vi "PC_TDVM_Single.vi"() -> ()   [LabVIEW 2021]
uses:
  Time Domain Measurement/Typedefs/Time Domain Measurements.ctl
  Time Domain Measurement/Typedefs/Timing & Trigger Settings.ctl
  Time Domain Measurement/Typedefs/Timing Settings.ctl
  Time Domain Measurement/Typedefs/Trigger Settings.ctl
  Time Domain Measurement/DAQ_Time Domain Measurement.lvlib
panel:
  out "Time Domain Measurements":T1={"Mean DC Voltage (V)"=[1.1069459616870432], "Vpp Amplitude(V)"=[5.075915353058466], "Voltage Frequency(Hz)"=[101.01007488404397], "Voltage Waveform Period (s)"=[0.009900002560615512], "Voltage Waveform duty cycle (%)"=[22.01996744294479]} {"Voltage Waveform duty cycle (%)" format="%.2p"; "Voltage Waveform Period (s)" format="%.2p"; "Voltage Frequency(Hz)" format="%.2p"; "Vpp Amplitude(V)" format="%.2p"; "Mean DC Voltage (V)" format="%.2p"}
  out "error out":errorcluster
  out "Voltage Waveforms":waveform(dbl)[](graph)=[{"t0"=timestamp(3797419317.779368 s since 1904-01-01), "dt"=9.999999999999972e-06, "Y"=array[10000 elements], "attributes"=variant("NI_ChannelName"=variant(string "Dev1/ai2"), "NI_UnitDescription"=variant(string "Volts"))}]
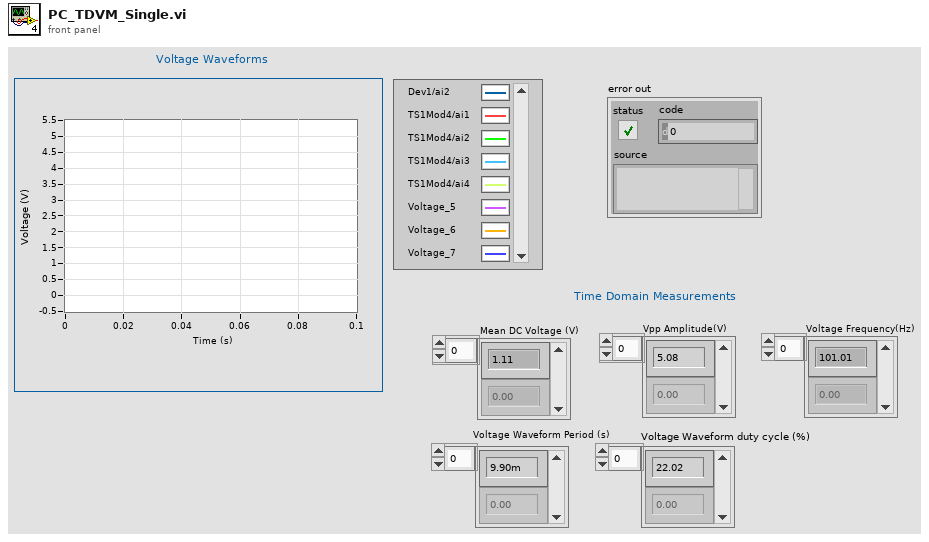
[diagram p1: front panel]
types:
  T1 = typedef "DAQ_Time Domain Measurement.lvlib/Time Domain Measurements.ctl" = cluster{"Mean DC Voltage (V)":dbl[], "Vpp Amplitude(V)":dbl[], "Voltage Frequency(Hz)":dbl[], "Voltage Waveform Period (s)":dbl[], "Voltage Waveform duty cycle (%)":dbl[]}
  T2 = typedef "DAQ_Time Domain Measurement.lvlib/Timing & Trigger Settings.ctl" = cluster{"Timing Settings":T3, "Trigger Settings":T4}
  T3 = typedef "DAQ_Time Domain Measurement.lvlib/Timing Settings.ctl" = cluster{"Sample Clock Source":tag, "Sample Rate(Hz)":dbl, "Number of Samples":i32, "Sample Timing Engine":enum16{"te0", "te1", "ai", "Auto"}}
  T4 = typedef "DAQ_Time Domain Measurement.lvlib/Trigger Settings.ctl" = cluster{"Trigger Type":enum16{"No Trigger", "Digital Start"}, "Digital Start Trigger Source":tag, "Digital Start Trigger Edge":i32}
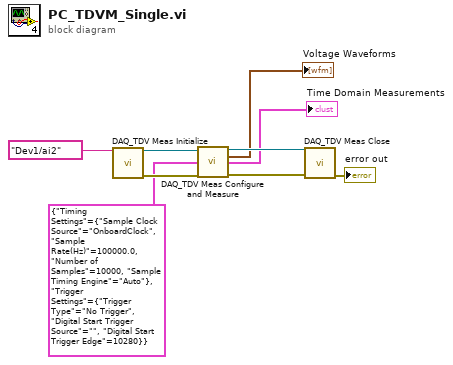
[diagram p0: block diagram]
diagram:
  n1 = call "DAQ_TDV Meas Initialize.vi"("Physical Channels"=tag "Dev1/ai2") -> ("DAQmx Task Out"=w9:refnum<k21>, "error out"=w8:errorcluster)  [unwired: 13 in]
  n2 = call "DAQ_TDV Meas Configure and Measure.vi"("DAQmx Task In"=w9, "Timing and Trigger Settings"=T2 {"Timing Settings"={"Sample Clock Source"="OnboardClock", "Sample Rate(Hz)"=100000.0, "Number of Samples"=10000, "Sample Timing Engine"=enum."Auto"}, "Trigger Settings"={"Trigger Type"=enum."No Trigger", "Digital Start Trigger Source"="", "Digital Start Trigger Edge"=10280}}, "error in"=w8) -> ("DAQmx Task Out"=w7:refnum<k21>, "Voltage Waveforms"=→"Voltage Waveforms":waveform(dbl)[], "Time Domain Measurements"=→"Time Domain Measurements":T1, "error out"=w6:errorcluster)  [unwired: 8 in, 1 out]
  n3 = call "DAQ_TDV Meas Close.vi"("DAQmx Task In"=w7, "error in"=w6) -> ("error out"=→"error out":errorcluster)  [unwired: 13 in]
